vi "datascopes.to_json.vi"(8 "error in":errorcluster, 10 "datascopes":T1) -> (0 "error out":errorcluster, 2 "json":string)   [LabVIEW 2020, in "nominal types.lvlib" / "dataScopes.lvlib"]
uses:
  dataScopes.lvlib
  data_scopes.ctl
  data_scope.ctl
  properties/properties.lvclass
  data_source.ctl
  type.ctl
  offset.ctl
  <vilib>/JDP Science/JSONtext/support/Format JSON Array Text.vi
  <vilib>/JDP Science/JSONtext/JSONtext.lvlib
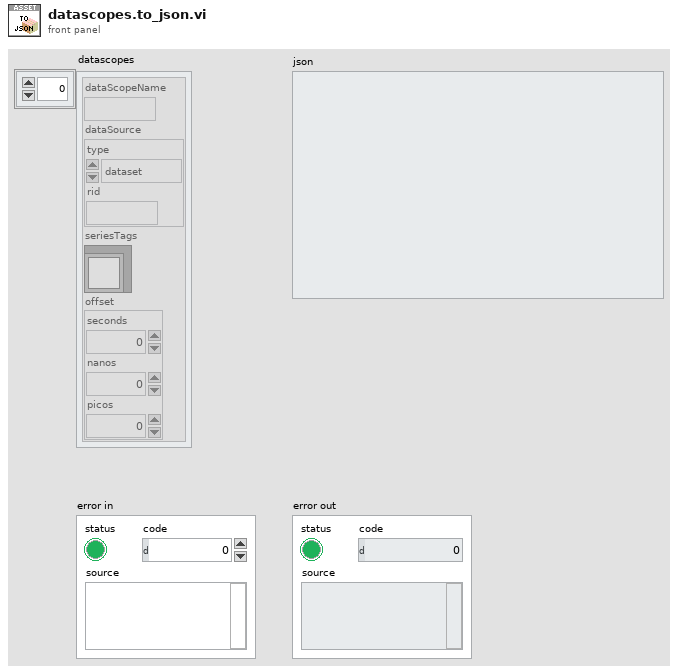
[diagram p1: front panel]
types:
  T1 = typedef "nominal types.lvlib/dataScopes.lvlib/data_scopes.ctl" = T2[]
  T2 = typedef "nominal types.lvlib/dataScopes.lvlib/data_scope.ctl" = cluster{"dataScopeName":string, "dataSource":T3, "seriesTags":refnum<class "properties.lvclass">, "offset":T5}
  T3 = typedef "nominal types.lvlib/dataScopes.lvlib/data_source.ctl" = cluster{"type":T4, "rid":string}
  T4 = typedef "nominal types.lvlib/dataScopes.lvlib/type.ctl" = enum16{"dataset", "connection", "logSet", "video"}
  T5 = typedef "nominal types.lvlib/dataScopes.lvlib/offset.ctl" = cluster{"seconds":i32, "nanos":i32, "picos":i32}
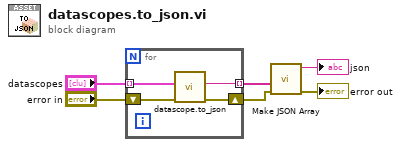
[diagram p0: block diagram]
diagram:
  n1 = for {
    tunnel: "datascopes" -> [w10] mode=indexing
    tunnel: [w9] -> w5 mode=indexing
    shift-right: [w8] -> w3
    shift-left: "error in" -> [w7]
    n2 = call "datascope.to_json.vi"("error in"=w7, "data scope"=w10) -> ("error out"=w8:errorcluster, "json"=w9:string)  [unwired: 8 in]
  }
  n3 = call <vilib>:"Make JSON Array.vi"("error in (no error)"=w3, "JSON Elements"=w5) -> ("error out"=→"error out":errorcluster, "<JSON>"=→"json":string)  [unwired: 8 in]
